vi "writeMotor.vi"(0 "Position":fxp<+/-,32,16>, 1 "Velocity":fxp<+/-,32,16>, 2 "Torque":fxp<+/-,32,16>, 3 "Kp":fxp<+/-,32,16>, 4 "Kd":fxp<+/-,32,16>, 5 "ID":u32 format="%x", 8 "SPI Config In":T1) -> (9 "SPI Config Out":T1)   [LabVIEW 2019]
uses:
  SPI/SPI Config.ctl
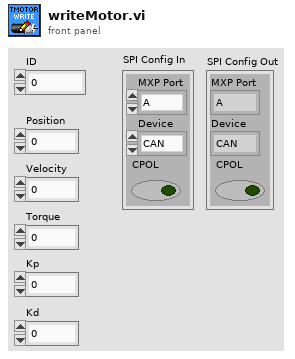
[diagram p1: front panel]
types:
  T1 = typedef "SPI Config.ctl" = cluster{"MXP Port":enum16{"A", "B"}, "Device":enum16{"CAN", "ENC", "IMU1", "IMU2"}, "CPOL":bool}
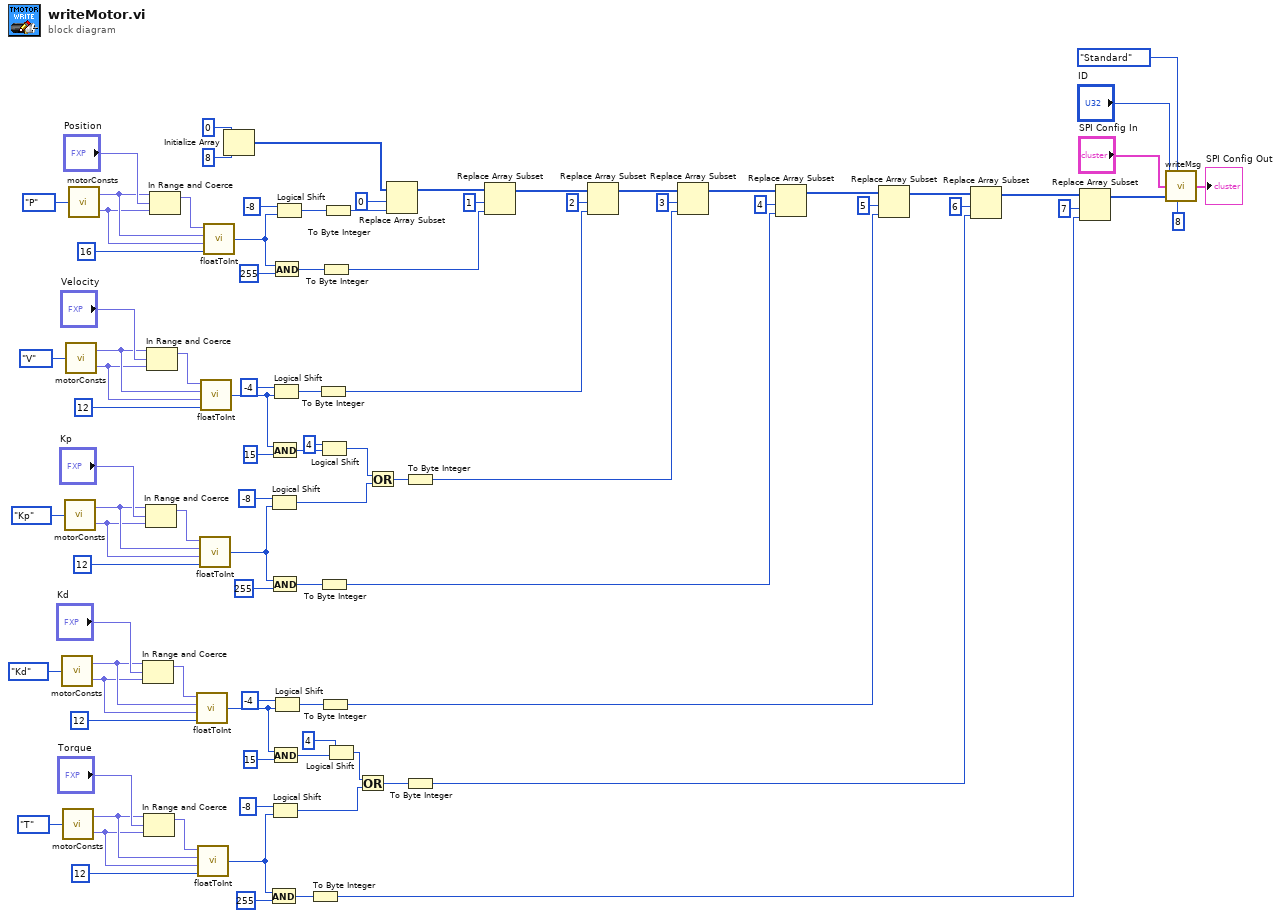
[diagram p0: block diagram]
diagram:
  n1 = call "motorConsts.vi"("Parameter"=enum16{"P", "V", "T", "Kp", "Kd"}."Kd" ("Enum")) -> ("Max"=w74:fxp<+/-,32,16>, "Min"=w73:fxp<+/-,32,16>)
  n2 = call "motorConsts.vi"("Parameter"=enum16{"P", "V", "T", "Kp", "Kd"}."T" ("Enum")) -> ("Max"=w68:fxp<+/-,32,16>, "Min"=w67:fxp<+/-,32,16>)
  n3 = call "motorConsts.vi"("Parameter"=enum16{"P", "V", "T", "Kp", "Kd"}."Kp" ("Enum")) -> ("Max"=w80:fxp<+/-,32,16>, "Min"=w79:fxp<+/-,32,16>)
  n4 = call "motorConsts.vi"("Parameter"=enum16{"P", "V", "T", "Kp", "Kd"}."V" ("Enum")) -> ("Max"=w86:fxp<+/-,32,16>, "Min"=w85:fxp<+/-,32,16>)
  n5 = call "motorConsts.vi"("Parameter"=enum16{"P", "V", "T", "Kp", "Kd"}."P" ("Enum")) -> ("Max"=w2:fxp<+/-,32,16>, "Min"=w1:fxp<+/-,32,16>)
  n6 = In Range and Coerce(upper limit=w74, x="Kd", lower limit=w73) -> (coerced(x)=w75:fxp<+/-,32,16>)  [unwired: 1 out]
  n7 = In Range and Coerce(upper limit=w68, x="Torque", lower limit=w67) -> (coerced(x)=w69:fxp<+/-,32,16>)  [unwired: 1 out]
  n8 = In Range and Coerce(upper limit=w80, x="Kp", lower limit=w79) -> (coerced(x)=w81:fxp<+/-,32,16>)  [unwired: 1 out]
  n9 = In Range and Coerce(upper limit=w86, x="Velocity", lower limit=w85) -> (coerced(x)=w87:fxp<+/-,32,16>)  [unwired: 1 out]
  n10 = In Range and Coerce(upper limit=w2, x="Position", lower limit=w1) -> (coerced(x)=w91:fxp<+/-,32,16>)  [unwired: 1 out]
  n11 = call "floatToInt.vi"("bits"=i16 12, "x_min"=w73, "x_max"=w74, "x"=w75) -> ("Integer"=w23:u32)
  n12 = call "floatToInt.vi"("bits"=i16 12, "x_min"=w67, "x_max"=w68, "x"=w69) -> ("Integer"=w12:u32)
  n13 = call "floatToInt.vi"("bits"=i16 12, "x_min"=w79, "x_max"=w80, "x"=w81) -> ("Integer"=w34:u32)
  n14 = call "floatToInt.vi"("bits"=i16 12, "x_min"=w85, "x_max"=w86, "x"=w87) -> ("Integer"=w47:u32)
  n15 = call "floatToInt.vi"("bits"=i16 16, "x_min"=w1, "x_max"=w2, "x"=w91) -> ("Integer"=w57:u32)
  n16 = Initialize Array(i8 0 ("element"), 8 ("dimension size")) -> (w61:i8[])
  n17 = Logical Shift(y=i16 -8, x=w34) -> (x << y=w41:u32)
  n18 = And(x=w12, y=u16 255) -> (x .and. y?=w10:u32)
  n19 = And(x=w47, y=u16 15) -> (x .and. y?=w45:u32)
  n20 = And(x=w34, y=u16 255) -> (x .and. y?=w32:u32)
  n21 = Logical Shift(y=i16 -8, x=w12) -> (x << y=w17:u32)
  n22 = Logical Shift(y=i16 -4, x=w47) -> (x << y=w49:u32)
  n23 = And(x=w23, y=u16 15) -> (x .and. y?=w21:u32)
  n24 = And(x=w57, y=u16 255) -> (x .and. y?=w55:u32)
  n25 = Logical Shift(y=i16 -4, x=w23) -> (x << y=w27:u32)
  n26 = Logical Shift(y=i16 -8, x=w57) -> (x << y=w64:u32)
  n27 = To Byte Integer(number=w10) -> (8bit integer=w9:i8)
  n28 = To Byte Integer(number=w49) -> (8bit integer=w48:i8)
  n29 = Logical Shift(y=i16 4, x=w45) -> (x << y=w42:u32)
  n30 = To Byte Integer(number=w32) -> (8bit integer=w31:i8)
  n31 = To Byte Integer(number=w27) -> (8bit integer=w26:i8)
  n32 = To Byte Integer(number=w55) -> (8bit integer=w53:i8)
  n33 = To Byte Integer(number=w64) -> (8bit integer=w59:i8)
  n34 = Logical Shift(y=i16 4, x=w21) -> (x << y=w18:u32)
  n35 = Or(x=w18, y=w17) -> (x .or. y?=w16:u32)
  n36 = Or(x=w42, y=w41) -> (x .or. y?=w38:u32)
  n37 = Replace Array Subset(array=w61, new element=w59, index=0) -> (w58:i8[])
  n38 = To Byte Integer(number=w38) -> (8bit integer=w37:i8)
  n39 = To Byte Integer(number=w16) -> (8bit integer=w15:i8)
  n40 = Replace Array Subset(array=w58, new element=w53, index=1) -> (w52:i8[])
  n41 = Replace Array Subset(array=w52, new element=w48, index=2) -> (w40:i8[])
  n42 = Replace Array Subset(array=w40, new element=w37, index=3) -> (w36:i8[])
  n43 = Replace Array Subset(array=w36, new element=w31, index=4) -> (w30:i8[])
  n44 = Replace Array Subset(array=w30, new element=w26, index=5) -> (w25:i8[])
  n45 = Replace Array Subset(array=w25, new element=w15, index=6) -> (w14:i8[])
  n46 = Replace Array Subset(array=w14, new element=w9, index=7) -> (w8:i8[])
  n47 = call "writeMsg.vi"("ID"="ID", "ID Type"=enum16{"Standard", "Extended"}."Standard", "SPI Config In"="SPI Config In", "Data to Write"=w8, "Frames to Write"=u8 8) -> ("SPI Config Out"=→"SPI Config Out":T1)
